vi "createDeviceData.vi"(8 "error in (no error)":errorcluster, 11 "RfOutputData in":refnum<class "RfOutputData.lvclass">) -> (0 "error out":errorcluster, 3 "RfOutputData out":refnum<class "RfOutputData.lvclass">)   [LabVIEW 2009, in "DataMappers.lvlib" / "RfOutputData.lvclass"]
uses:
  RfOutputData.lvclass
  Hal/Channels/DDSOutput/Generic/DDSOutput.lvclass
  RfOutputData.lvclass/RfOutputData.ctl
  DeviceData.lvclass
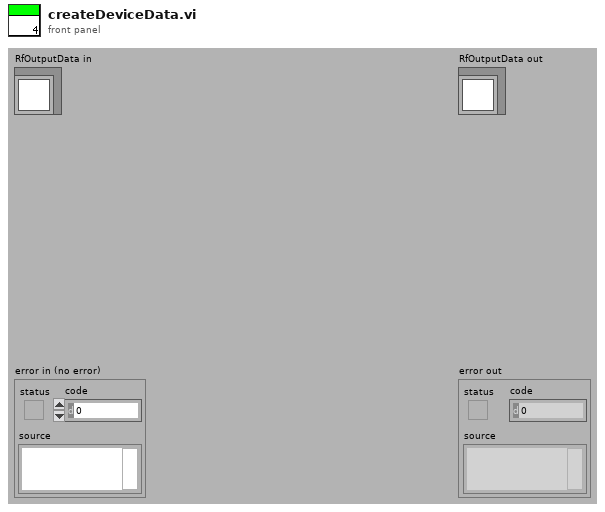
[diagram p1: front panel]
types:
  T1 = cluster{"OutputForm":enum16{"Sine", "Square", "Triangle", "Arbitrary"}[], "OutputFunction":enum16{"Frequency", "Ramp", "Sequence"}[], "physicalChannels":string}
  T2 = cluster{"freq":dbl, "Amp":dbl, "phase":dbl, "time":dbl, "RfChannel":refnum<class "RfOutputChannel.lvclass">}[][]
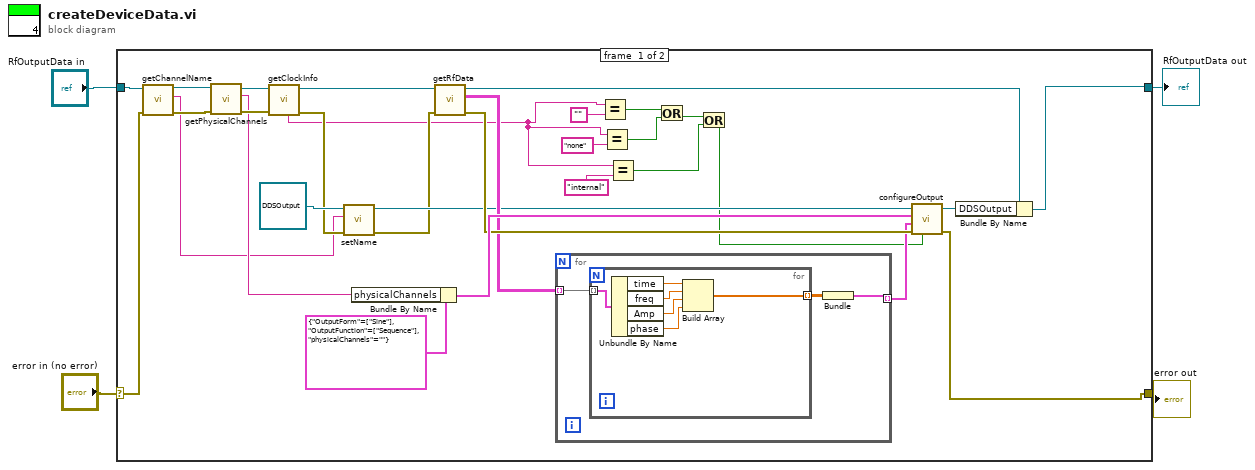
[diagram p0: block diagram]
diagram:
  n1 = case shown="No Error" "error in (no error)" {
    selector: "error in (no error)" -> [w20 w45]
    tunnel: [w25 w45] -> w3
    tunnel: [w26 w46] -> w2
    tunnel: "RfOutputData in" -> [w21 w46]
    frame #0 {
      n2 = call "getChannelName.vi"("error in (no error)"=w20, "DeviceData in"=w21) -> ("error out"=w19:errorcluster, "channelName"=w14:string, "DeviceData out"=w22:refnum<class "RfOutputData.lvclass">)  [unwired: 7 in]
      n3 = call "getPhysicalChannels.vi"("error in (no error)"=w19, "DeviceData in"=w22) -> ("error out"=w34:errorcluster, "physicalChannels"=w33:string, "DeviceData out"=w35:refnum<class "RfOutputData.lvclass">)  [unwired: 7 in]
      n4 = call "getClockInfo.vi"("error in (no error)"=w34, "DeviceData in"=w35) -> ("error out"=w16:errorcluster, "DeviceData out"=w30:refnum<class "RfOutputData.lvclass">, "start_trigger"=w8:string)  [unwired: 5 in, 2 out]
      n5 = call "setName.vi"("error in (no error)"=w16, "name"=w14, "DDSOutput in"=refnum<class "DDSOutput.lvclass"> refnum) -> ("error out"=w15:errorcluster, "DDSOutput out"=w17:refnum<class "DDSOutput.lvclass">)  [unwired: 7 in]
      n6 = Bundle By Name(cluster=T1 {"OutputForm"=[enum."Sine"], "OutputFunction"=[enum."Sequence"], "physicalChannels"=""} ("Config"), "physicalChannels"=w33) -> (w32:T1)
      n7 = call "getRfData.vi"("error in (no error)"=w15, "RfOutputData in"=w30) -> ("error out"=w29:errorcluster, "rfData"=w24:T2, "RfOutputData out"=w28:refnum<class "RfOutputData.lvclass">)  [unwired: 7 in]
      n8 = for {
        tunnel: w24 -> [w38] mode=indexing
        tunnel: [w36] -> w23 mode=indexing
        n9 = for {
          tunnel: w38 -> [w44] mode=indexing
          tunnel: [w39] -> w37 mode=indexing
          n10 = Unbundle By Name(w44) -> ("time"=w43:dbl, "freq"=w42:dbl, "Amp"=w41:dbl, "phase"=w40:dbl)
          n11 = Build Array(w43, w42, w41, w40) -> (w39:dbl[])
        }
        n12 = Bundle(w37) -> (w36:cluster{dbl[][]})  [unwired: 1 in]
      }
      n13 = Equal?(x=w8, y="") -> (x = y?=w11:bool)
      n14 = Equal?(x=w8, y="none") -> (x = y?=w10:bool)
      n15 = Equal?(x=w8, y="internal") -> (x = y?=w6:bool)
      n16 = Or(x=w11, y=w10) -> (x .or. y?=w9:bool)
      n17 = Or(x=w9, y=w6) -> (x .or. y?=w5:bool)
      n18 = call-dynamic "configureOutput.vi"("sofwareTrigger?"=w5, "error in (no error)"=w29, "Data"=w23, "Config"=w32, "DDSOutput in"=w17) -> ("error out"=w25:errorcluster, "DDSOutput out"=w27:refnum<class "DDSOutput.lvclass">)  [unwired: 5 in]
      n19 = Bundle By Name(cluster=w28, "DDSOutput"=w27) -> (w26:refnum<class "RfOutputData.lvclass">)
    }
    frame #1 {
    }
  }
  "error out" <- w3
  "RfOutputData out" <- w2
